vi "rms.vi"() -> ()   [LabVIEW 2015]
uses:
  <vilib>/Analysis/5stat.llb/RMS (DBL).vi
  <vilib>/Analysis/NI_AALPro.lvlib
panel:
  out "rms value":dbl format="%0.2f"
  out "number":i32
  out "substring before match":string
  out "Array 2":string[](array[string])
  out "substring":string
  out "length":i32
  in  "String":string
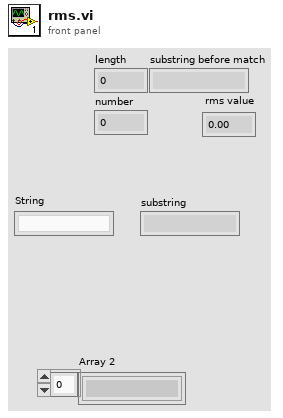
[diagram p1: front panel]
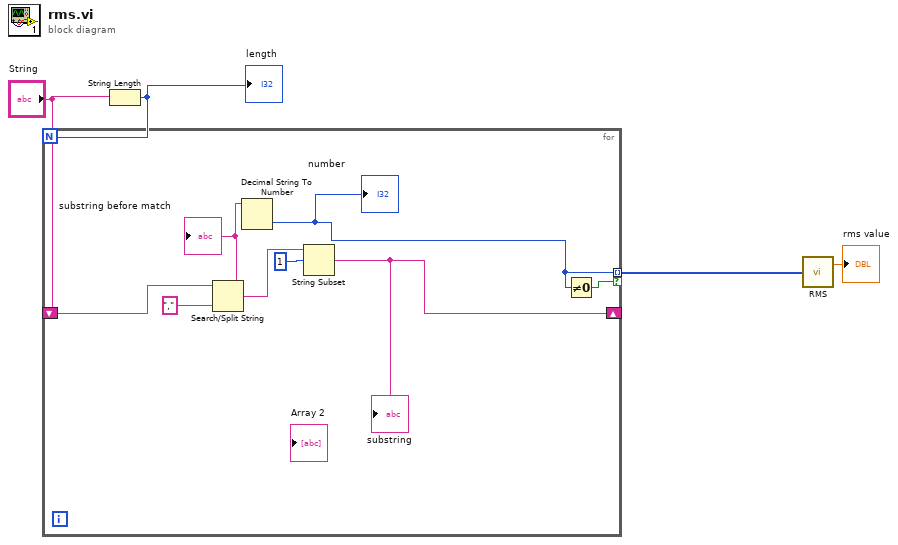
[diagram p0: block diagram]
diagram:
  n1 = String Length(string="String") -> (length=w4:i32)
  "length" <- w4
  n2 = for {
    N: w4 -> [_]
    shift-right: [w8] -> _
    shift-left: "String" -> [w11]
    tunnel: [w5] -> w2 mode=indexing if=w6
    n3 = Search/Split String(string=w11, search string/char (-)=",") -> (substring before match=w7:string, match + rest of string=w10:string)  [unwired: 1 in, 1 out]
    "substring before match" <- w7
    n4 = Decimal String To Number(string=w7) -> (number=w5:i32)  [unwired: 2 in, 1 out]
    "number" <- w5
    n5 = String Subset(string=w10, offset (0)=1) -> (substring=w8:string)  [unwired: 1 in]
    "substring" <- w8
    n6 = Not Equal To 0?(x=w5) -> (x != 0?=w6:bool)
  }
  n7 = call-poly <vilib>:"RMS.vi"("X"=w2) -> ("rms value"=→"rms value":dbl)  [unwired: 1 out]
